vi "setTriggerIndicatorVisible.vi"(10 "NewVal":T1, 11 "Trigger ref":refnum<vi>[](array[refnum])) -> ()   [LabVIEW 2013]
uses:
  Device Drivers/PXIdigitizer/mode_TypDef.ctl
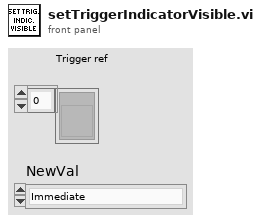
[diagram p1: front panel]
types:
  T1 = typedef "mode_TypDef.ctl" = enum32{"Immediate", "Analog Edge", "Analog Window", "Analog Hysteresis", "Video", "Digital Edge"}
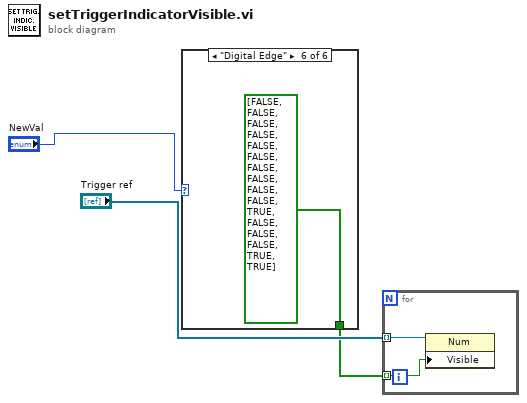
[diagram p0: block diagram]
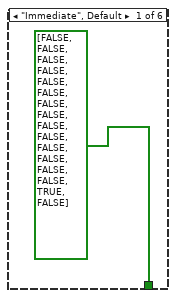
[diagram p2: hidden frame]
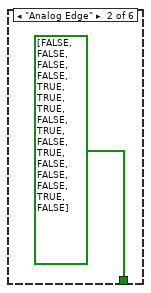
[diagram p3: hidden frame]
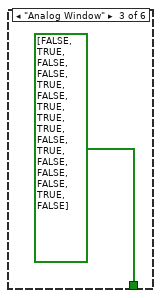
[diagram p4: hidden frame]
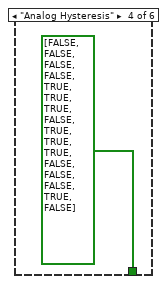
[diagram p5: hidden frame]
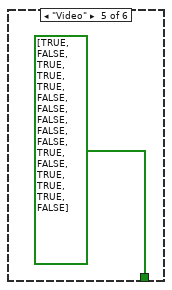
[diagram p6: hidden frame]
diagram:
  n1 = case shown="\"Digital Edge\"" "NewVal" {
    tunnel: [bool[] [FALSE, FALSE, FALSE, FALSE, FALSE, FALSE, FALSE, FALSE, FALSE, FALSE, FALSE, FALSE, FALSE, FALSE, TRUE, FALSE] bool[] [FALSE, FALSE, FALSE, FALSE, TRUE, TRUE, TRUE, FALSE, TRUE, FALSE, TRUE, FALSE, FALSE, FALSE, TRUE, FALSE] bool[] [FALSE, TRUE, FALSE, FALSE, TRUE, FALSE, TRUE, TRUE, TRUE, FALSE, TRUE, FALSE, FALSE, FALSE, TRUE, FALSE] bool[] [FALSE, FALSE, FALSE, FALSE, TRUE, TRUE, TRUE, FALSE, TRUE, TRUE, TRUE, FALSE, FALSE, FALSE, TRUE, FALSE] bool[] [TRUE, FALSE, TRUE, TRUE, TRUE, FALSE, FALSE, FALSE, FALSE, FALSE, TRUE, FALSE, TRUE, TRUE, TRUE, FALSE] bool[] [FALSE, FALSE, FALSE, FALSE, FALSE, FALSE, FALSE, FALSE, FALSE, FALSE, TRUE, FALSE, FALSE, FALSE, TRUE, TRUE]] -> w1
    frame "Immediate", Default {
    }
    frame "Analog Edge" {
    }
    frame "Analog Window" {
    }
    frame "Analog Hysteresis" {
    }
    frame "Video" {
    }
    frame "Digital Edge" {
    }
  }
  n2 = for {
    tunnel: "Trigger ref" -> [w11] mode=indexing
    tunnel: w1 -> [w10] mode=indexing
    n3 = property class="Num"(reference=w11, "Visible"=w10) -> ()  [unwired: 1 in, 2 out]
  }
